vi "NumberCheckMarcoGonzalez.vi"() -> ()   [LabVIEW 2012]
doc: "This VI will generate a one dimensional array with 10 elements filled with random integers and a number check of this array. The inputs should be an upper range (0 will be at the bottom) for the random integer array and an integer that will serve as the check. The ouputs will be the numeric array and a check array."
panel:
  out "Check Array":dbl[](array[numeric])
  in  "Check Integer":dbl
  in  "Range (From 0)":dbl
  out "Numeric Array":dbl[](array[numeric])
  # "Marco Gonzalez\nEA3\n03 / 14 / 2017"
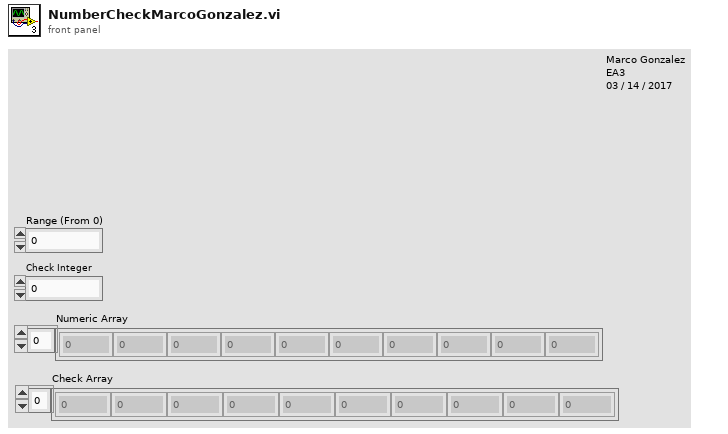
[diagram p1: front panel]
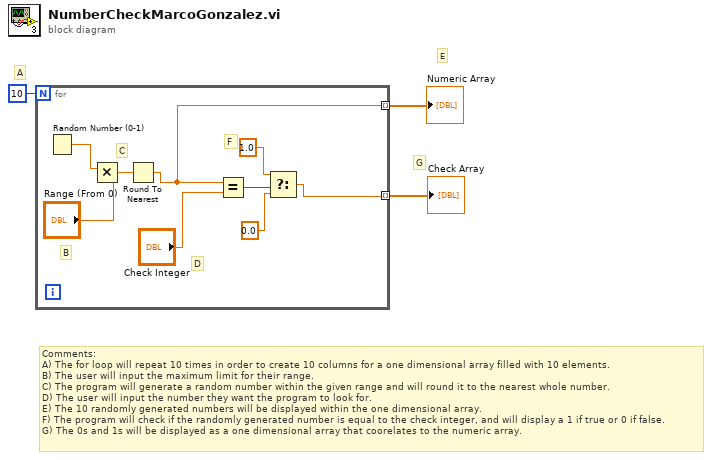
[diagram p0: block diagram]
diagram:
  # "Comments:\nA) The for loop will repeat 10 times in order to create 10 columns for a one dimensional array filled with 10 elements.\nB) The user will input the maximum limit for their range.\nC) The program will generate a random number within the given range and will round it to the nearest whole number.\nD) The user will input the number they want the program to look for.\nE) The 10 randomly generated numbers will be displayed within the one dimensional array. \nF) The program will check if the randomly generated number is equal to the check integer, and will display a 1 if true or 0 if false.\nG) The 0s and 1s will be displayed as a one dimensional array that coorelates to the numeric array."
  # "G"
  # "E"
  # "A"
  n1 = for {
    N: 10 -> [_]
    tunnel: [w4] -> w2 mode=indexing
    tunnel: [w7] -> w1 mode=indexing
    # "F"
    # "D"
    # "B"
    # "C"
    n2 = Random Number (0-1)() -> (number: 0 to 1=w6:dbl)
    n3 = Multiply(x=w6, y="Range (From 0)") -> (x*y=w5:dbl)
    n4 = Round To Nearest(number=w5) -> (nearest integer value=w4:dbl)
    n5 = Equal?(x=w4, y="Check Integer") -> (x = y?=w11:bool)
    n6 = Select(t=1.0, s=w11, f=0.0) -> (s? t:f=w7:dbl)
  }
  "Numeric Array" <- w2
  "Check Array" <- w1
